vi "2100_Test_Butterfly.vi"(0 "Semiconductor Module Context":T6, 1 "Current  Level":dbl=0.01, 2 "Master_Register_Data_Array_In":T1 {"Address" format="%.0x"}, 5 "Script_Info":T4={"Script Name"="Butterfly", "All_Scripts"=[]}, 7 "Source Delay":dbl format="%#_6p", 9 "USID":T3 max=15, 11 "Error In":errorcluster, 12 "Instrument_Pins":T5={"SMU_Pins"=["RF1", "RF2", "RF3", "RF4"], "HSDIO_Pins"=["CLK", "SDA"]}, 13 "Thresholds(max R 1st)":dbl[](array[numeric])=[100000.0, 0.5], 14 "HV_Voltages":dbl[](array[numeric])) -> (6 "Master_Register_Data_Array_Out":T1 {"Address" format="%.0x"}, 15 "Error Out":errorcluster)   [LabVIEW 2013]
uses:
  Controls/USID.ctl
  <vilib>/NI_TestStand_SemiconductorModule/NI_TestStand_Semiconductor_Module.lvlibp/PinMap/General/SemiconductorModuleContext.ctl
  Controls/Master_Reg_Data_Array.ctl
  Controls/Reg_Address_Data.ctl
  <vilib>/NI_TestStand_SemiconductorModule/NI_TestStand_Semiconductor_Module.lvlibp/PinMap/General/Publish/PublishDataDoubleFunctionalTest.vi
  <vilib>/NI_TestStand_SemiconductorModule/NI_TestStand_Semiconductor_Module.lvlibp
panel:
  out "R Array":dbl[][](array[numeric])
  in  "Tab Control":enum32{"Test Info", "Instrument Settings"}(tab)
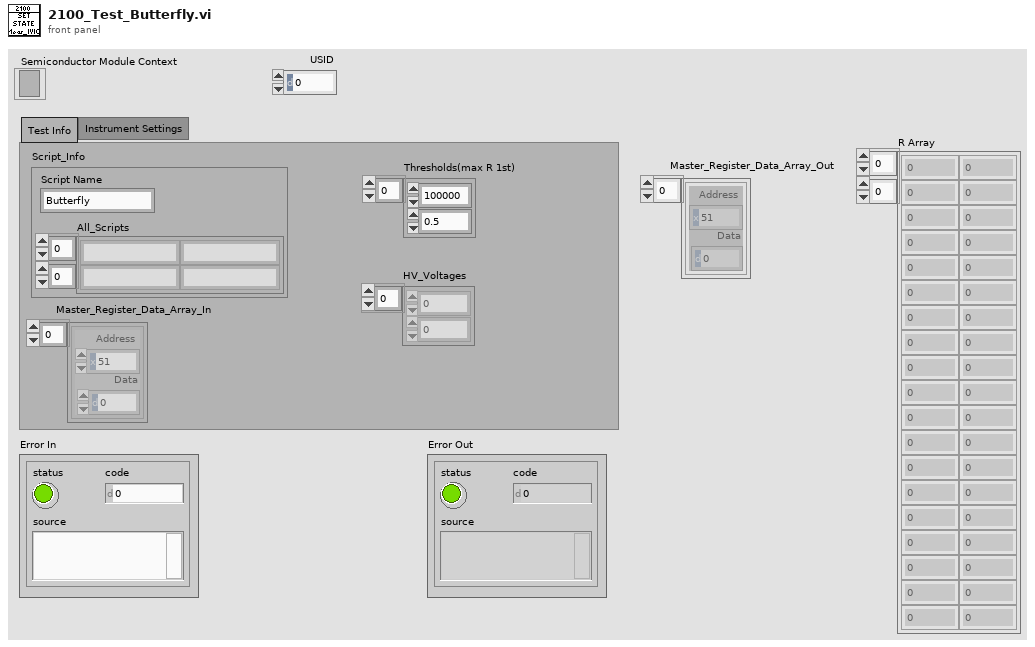
[diagram p1: front panel]
types:
  T1 = typedef "Master_Reg_Data_Array.ctl" = T2[]
  T2 = typedef "Reg_Address_Data.ctl" = cluster{"Address":u8, "Data":u8}
  T3 = typedef "USID.ctl" = u8
  T4 = cluster{"Script Name":string, "All_Scripts":string[][]}
  T5 = cluster{"SMU_Pins":string[], "HSDIO_Pins":string[]}
  T6 = typedef "NI_TestStand_Semiconductor_Module.lvlibp/SemiconductorModuleContext.ctl" = refnum<k7>
  T7 = typedef "Script Functions_Array.ctl" = enum16{"Reg_Write", "Bit_Write", "Delay", "Read", "Measure"}[]
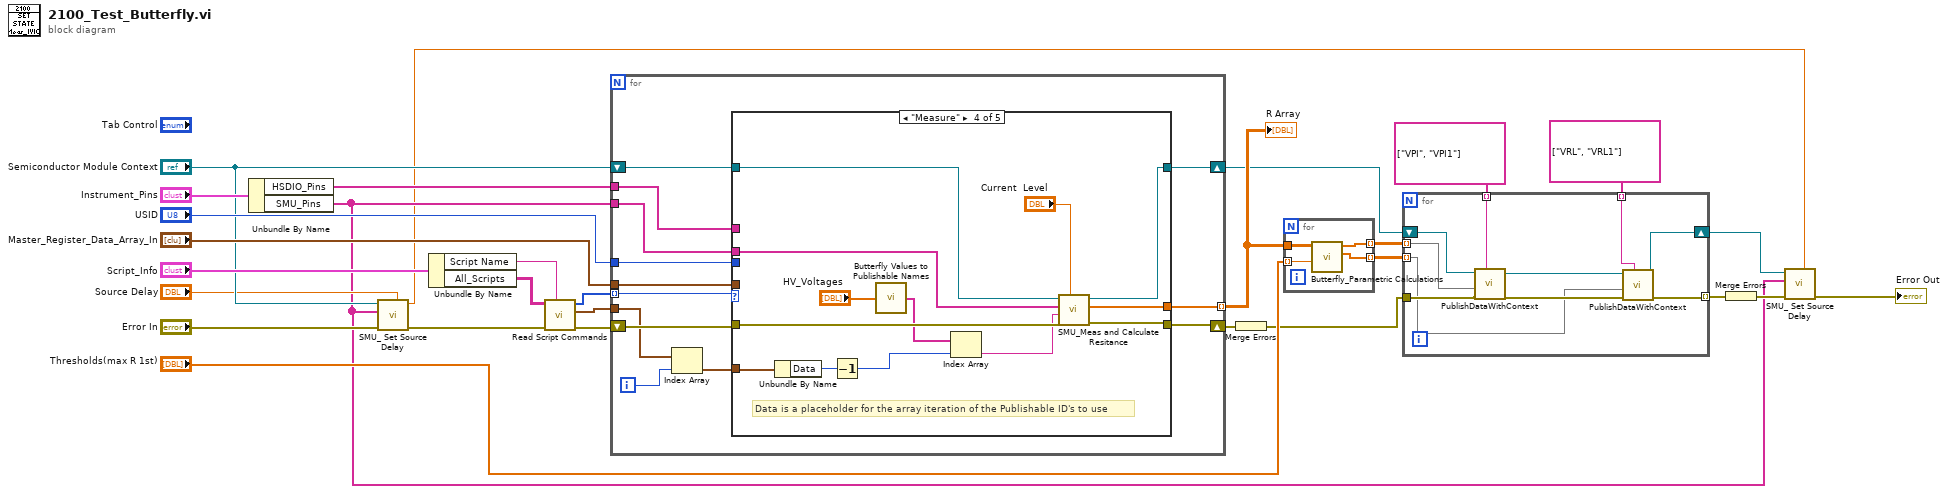
[diagram p0: block diagram]
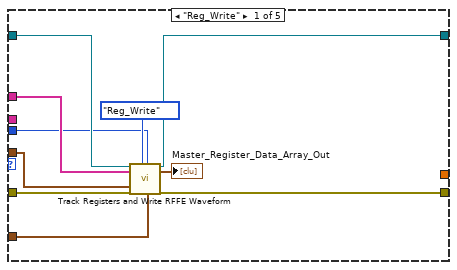
[diagram p2: hidden frame]
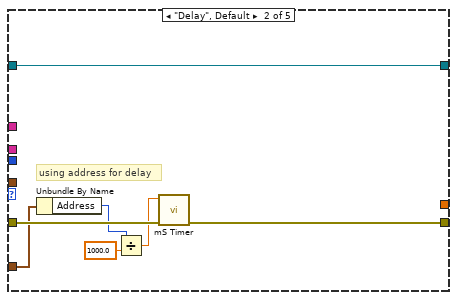
[diagram p3: hidden frame]
diagram:
  n1 = Unbundle By Name("Instrument_Pins") -> ("HSDIO_Pins"=w22:string[], "SMU_Pins"=w2:string[])
  n2 = call "SMU_ Set Source Delay.vi"("Source Delay"="Source Delay", "error in (no error)"="Error In", "Pins"=w2, "Semiconductor Module Context"="Semiconductor Module Context") -> ("error out"=w8:errorcluster, "Source Delay Readback"=w1:dbl)  [unwired: 6 in]
  n3 = Unbundle By Name("Script_Info") -> ("Script Name"=w19:string, "All_Scripts"=w20:string[][])
  n4 = call "Read Script Commands.vi"("Test Name"=w19, "Error In"=w8, "All_Scripts"=w20) -> ("Error Out"=w26:errorcluster, "Script_Data"=w27:T2[], "Script_Functions"=w28:T7)  [unwired: 5 in, 1 out]
  n5 = for {
    tunnel: "USID" -> [w36]
    tunnel: w28 -> [w35] mode=indexing
    tunnel: w27 -> [w39]
    tunnel: w22 -> [w40]
    shift-right: [w32] -> w24
    shift-left: w26 -> [w42]
    tunnel: "Master_Register_Data_Array_In" -> [w37]
    tunnel: w2 -> [w31]
    tunnel: [w33] -> w18 mode=indexing
    shift-right: [w30] -> w11
    shift-left: "Semiconductor Module Context" -> [w41]
    i -> [w34]
    n6 = Index Array(array=w39, index=w34) -> (element=w38:T2)
    n7 = case shown="\"Measure\"" w35 {
      tunnel: w38 -> [w47 w58 _ w70 _]
      tunnel: w42 -> [w52 w59 w61 w73 w76]
      tunnel: w36 -> [w44 _ _ _ _]
      tunnel: w41 -> [w50 w53 w60 w71 w75]
      tunnel: w40 -> [w49 _ _ _ _]
      tunnel: [w51 w57 w61 w74 w76] -> w32
      tunnel: w37 -> [w46 _ _ _ _]
      tunnel: [_ _ _ w72 _] -> w33
      tunnel: w31 -> [_ _ _ w66 _]
      tunnel: [w43 w53 w60 w62 w75] -> w30
      frame "Reg_Write" {
        n8 = call "Track Registers and Write RFFE Waveform.vi"("Semiconductor Module Context"=w50, "Pins"=w49, "Master_Register_Data_Array_In"=w46, "Error In"=w52, "Script_Functions"=enum16{"Reg_Write", "Bit_Write"}."Reg_Write", "USID"=w44, "Reg_Address_Data"=w47) -> ("Semiconductor Module Context Out"=w43:T6, "Master_Register_Data_Array_Out"=→"Master_Register_Data_Array_Out":T1, "Error Out"=w51:errorcluster)  [unwired: 10 in]
      }
      frame "Delay", Default {
        # "using address for delay"
        n9 = Unbundle By Name(w58) -> ("Address"=w55:u8)
        n10 = Divide(x=w55, y=1000.0) -> (x/y=w54:dbl)
        n11 = call "mS Timer.vi"("Error In"=w59, "Delay(S)"=w54) -> ("Error Out"=w57:errorcluster)  [unwired: 9 in]
      }
      frame "Read" {
      }
      frame "Measure" {
        # "Data is a placeholder for the array iteration of the Publishable ID's to use"
        n12 = Unbundle By Name(w70) -> ("Data"=w69:u8)
        n13 = Decrement(x=w69) -> (x-1=w68:u8)
        n14 = call "Butterfly Values to Publishable Names.vi"("Butterfly Numbers"="HV_Voltages") -> ("Publishable Names"=w63:string[])
        n15 = Index Array(array=w63, index=w68) -> (element=w67:string)
        n16 = call "SMU_Meas and Calculate Resitance.vi"("Current  Level"="Current  Level", "error in (no error)"=w73, "Published Data Id"=w67, "Pins"=w66, "Semiconductor Module Context"=w71) -> ("error Out"=w74:errorcluster, "R Array"=w72:dbl[], "Semiconductor Module Context Out"=w62:T6)  [unwired: 4 in]
      }
      frame "Bit_Write" {
      }
    }
  }
  "R Array" <- w18
  n17 = Merge Errors(w24) -> (w12:errorcluster)
  n18 = for {
    tunnel: w18 -> [w80]
    tunnel: [w79] -> w14 mode=indexing
    tunnel: [w78] -> w13 mode=indexing
    tunnel: "Thresholds(max R 1st)" -> [w77] mode=indexing
    n19 = call "Butterfly_Parametric Calculations.vi"("Threshold"=w77, "Result Array In"=w80) -> ("VRLs"=w78:dbl[], "VPIs"=w79:dbl[])  [unwired: 8 in]
  }
  n20 = for {
    tunnel: w12 -> [w90]
    tunnel: [w87] -> w10 mode=indexing
    tunnel: w14 -> [w85] mode=indexing
    tunnel: w13 -> [w82] mode=indexing
    tunnel: string[] ["VPI", "VPI1"] -> [w84] mode=indexing
    tunnel: string[] ["VRL", "VRL1"] -> [w83] mode=indexing
    shift-right: [w81] -> w3
    shift-left: w11 -> [w89]
    n21 = call-poly <vilib>:"PublishDataWithContext.vi"("Published Data Id"=w84, "error in (no error)"=w90, "Data In"=w85, "Semiconductor Module Context"=w89) -> ("error out"=w88:errorcluster, "Semiconductor Module Context Out"=w86:T6)  [unwired: 6 in]
    n22 = call-poly <vilib>:"PublishDataWithContext.vi"("Published Data Id"=w83, "error in (no error)"=w88, "Data In"=w82, "Semiconductor Module Context"=w86) -> ("error out"=w87:errorcluster, "Semiconductor Module Context Out"=w81:T6)  [unwired: 6 in]
  }
  n23 = Merge Errors(w10) -> (w5:errorcluster)
  n24 = call "SMU_ Set Source Delay.vi"("Source Delay"=w1, "error in (no error)"=w5, "Pins"=w2, "Semiconductor Module Context"=w3) -> ("error out"=→"Error Out":errorcluster)  [unwired: 6 in, 1 out]
